vi "Deselect Devices.vi"(8 "error in (no error)":errorcluster, 11 "DeviceListPanel in":refnum<class "DeviceListPanel.lvclass">) -> (0 "error out":errorcluster, 3 "DeviceListPanel out":refnum<class "DeviceListPanel.lvclass">)   [LabVIEW 2020, in "PicoG-App.lvlib" / "DeviceListPanel.lvclass"]
uses:
  DeviceListPanel.lvclass
  <vilib>/IlluminatedG/IG OOPanel/OOPanel/ArrayManager/ArrayManager.lvclass
  DeviceArrayPanel/DeviceArrayPanel.lvclass
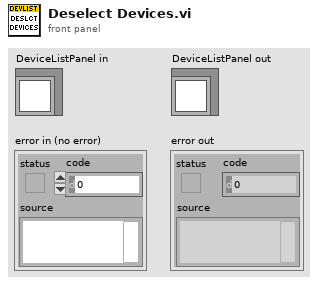
[diagram p1: front panel]
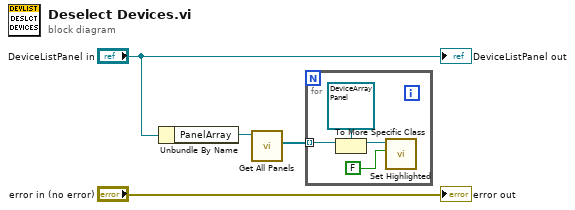
[diagram p0: block diagram]
diagram:
  n1 = Unbundle By Name("DeviceListPanel in") -> ("PanelArray"=w3:refnum<class "ArrayManager.lvclass">)
  n2 = call <vilib>:"Get All Panels.vi"("PanelArray in"=w3) -> ("Panels"=w1:refnum<class "ArrayPanel.lvclass">[])  [unwired: 8 in, 2 out]
  n3 = for {
    tunnel: w1 -> [w8] mode=indexing
    n4 = To More Specific Class(target class=refnum<class "DeviceArrayPanel.lvclass"> refnum ("PicoG-App.lvlib:DeviceArrayPanel.lvclass"), reference=w8) -> (specific class reference=w6:refnum<class "DeviceArrayPanel.lvclass">)  [unwired: 1 in, 1 out]
    n5 = call "Set Highlighted.vi"("Highlighted"=FALSE, "DeviceArrayPanel in"=w6) -> ()  [unwired: 8 in, 2 out]
  }
  "error out" <- "error in (no error)"
  "DeviceListPanel out" <- "DeviceListPanel in"
